vi "TCP.IP Client for Ripple Detection - Copy 5.vi"() -> ()   [LabVIEW 2021]
doc: "Demonstrates how to open a connection to an TCP server, read the data being sent, and display the data on a chart. This VI is designed to stop if the TCP connection is terminated."
uses:
  <vilib>/Utility/file.llb/Write To Spreadsheet File (string).vi
  <vilib>/Utility/file.llb/Write Delimited Spreadsheet (DBL).vi
  <vilib>/Utility/file.llb/Write To Spreadsheet File (DBL).vi
panel:
  in  "Header Info":string[][](table)=[["Test Name", "Operator", "UUT"], ["Voltage Test", "Nigel", "AAA123"]]
  in  "File Name":path=path "C:/Documents and Settings/husmith/Desktop/CSVdata.csv"
  in  "Channel Names":string[](array[string])=["Channel 1", "Channel 2", "Channel 3", "Channel 4", "Channel 5"]
  out "Filtered":dbl[](graph)
  out "Array Size 3":u32
  out "Delayed RMS2>RMS1 for 3 data":dynamicdata(graph)
  out "RMS2>RMS1 for 3 data":dynamicdata(graph)
  out "Array Size":u32
  out "RMS2>RMS1":dynamicdata(graph)
  out "RMS1":dynamicdata(graph)
  out "RMS2":dynamicdata(graph)
  out "Raw Data Collected":dynamicdata(graph)
  in  "Boolean":bool
  in  "Server Closed":string="The server VI closed the connection."
  out "Raw Data":dbl[](graph)
  in  "Stop":bool
  # "Overview: Demonstrates the use of the TCP functions to connect to a TCP server VI and receive data.\nInstructions:\n1. Ensure Simple TCP - Server.vi is already running.\n2. Run the VI.\n3. Click Stop to stop the VI. Note that if you stop the server VI, this VI will stop automatically."
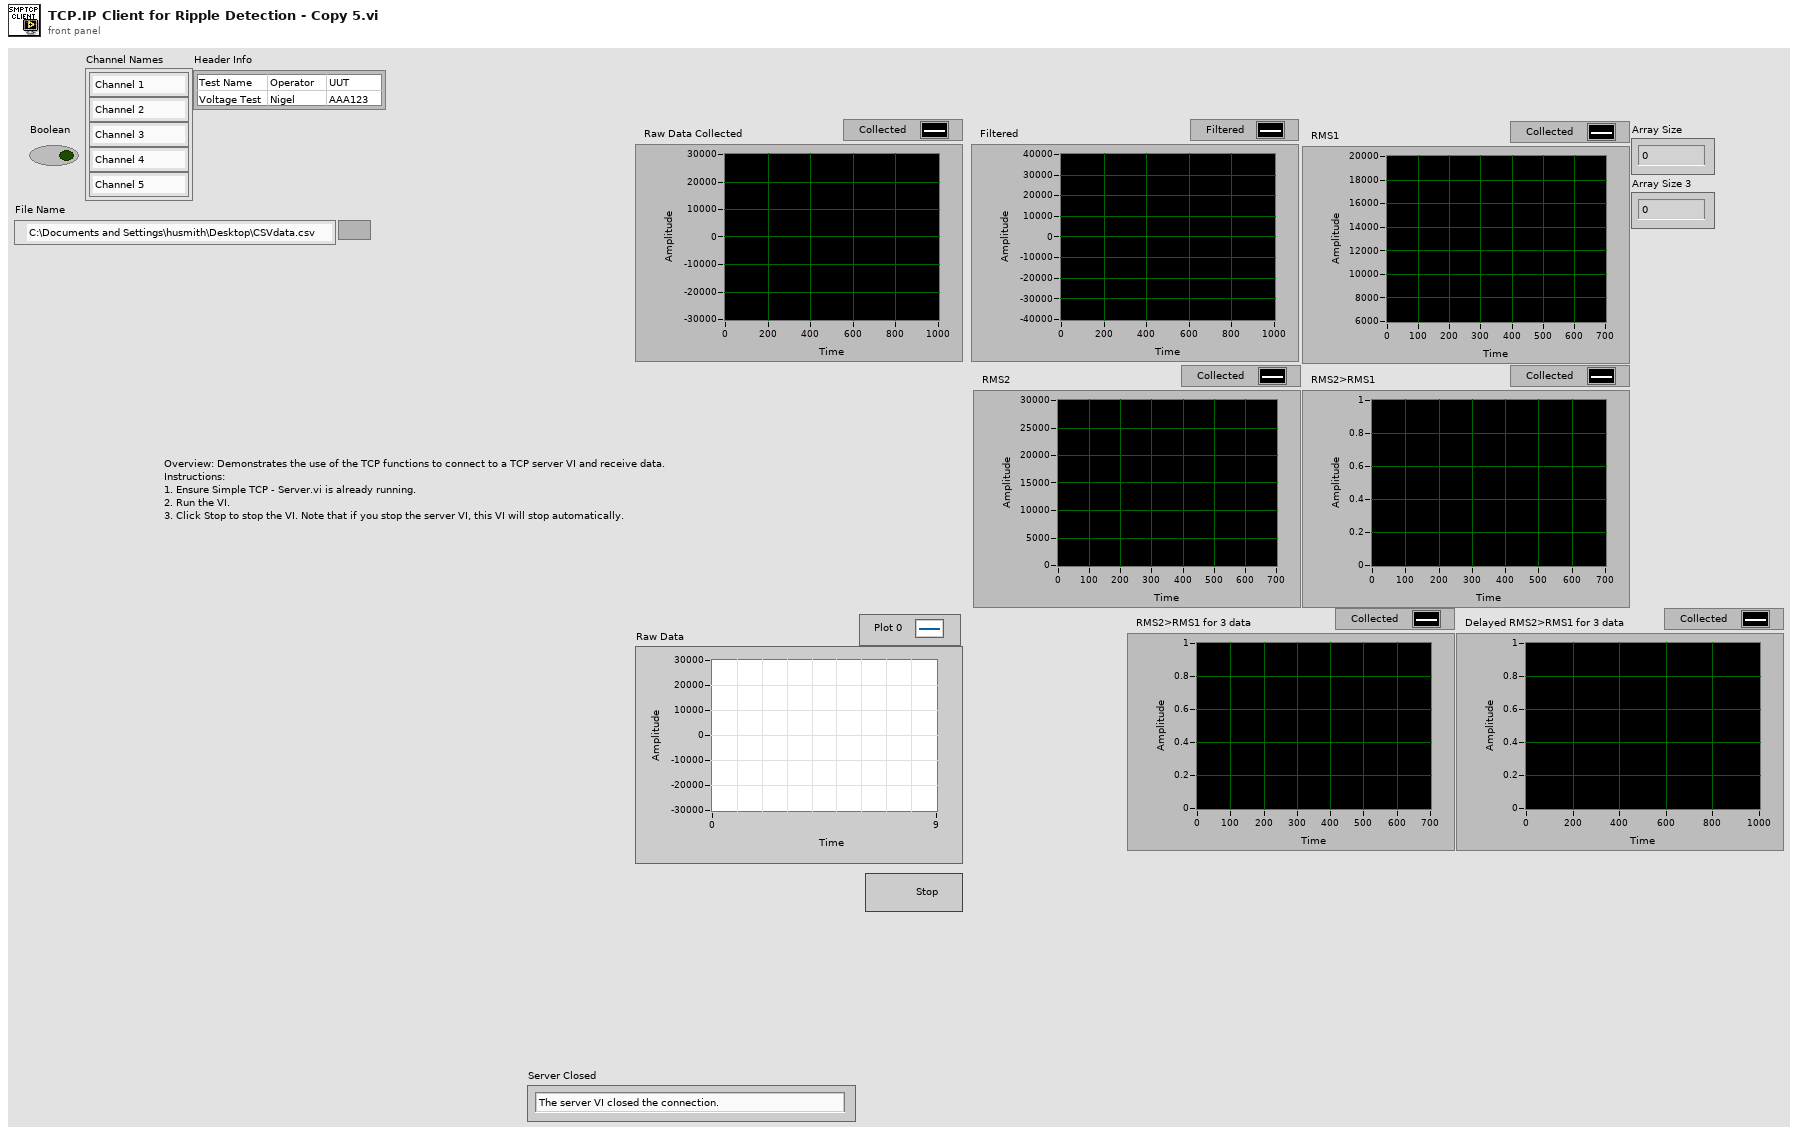
[diagram p1: front panel]
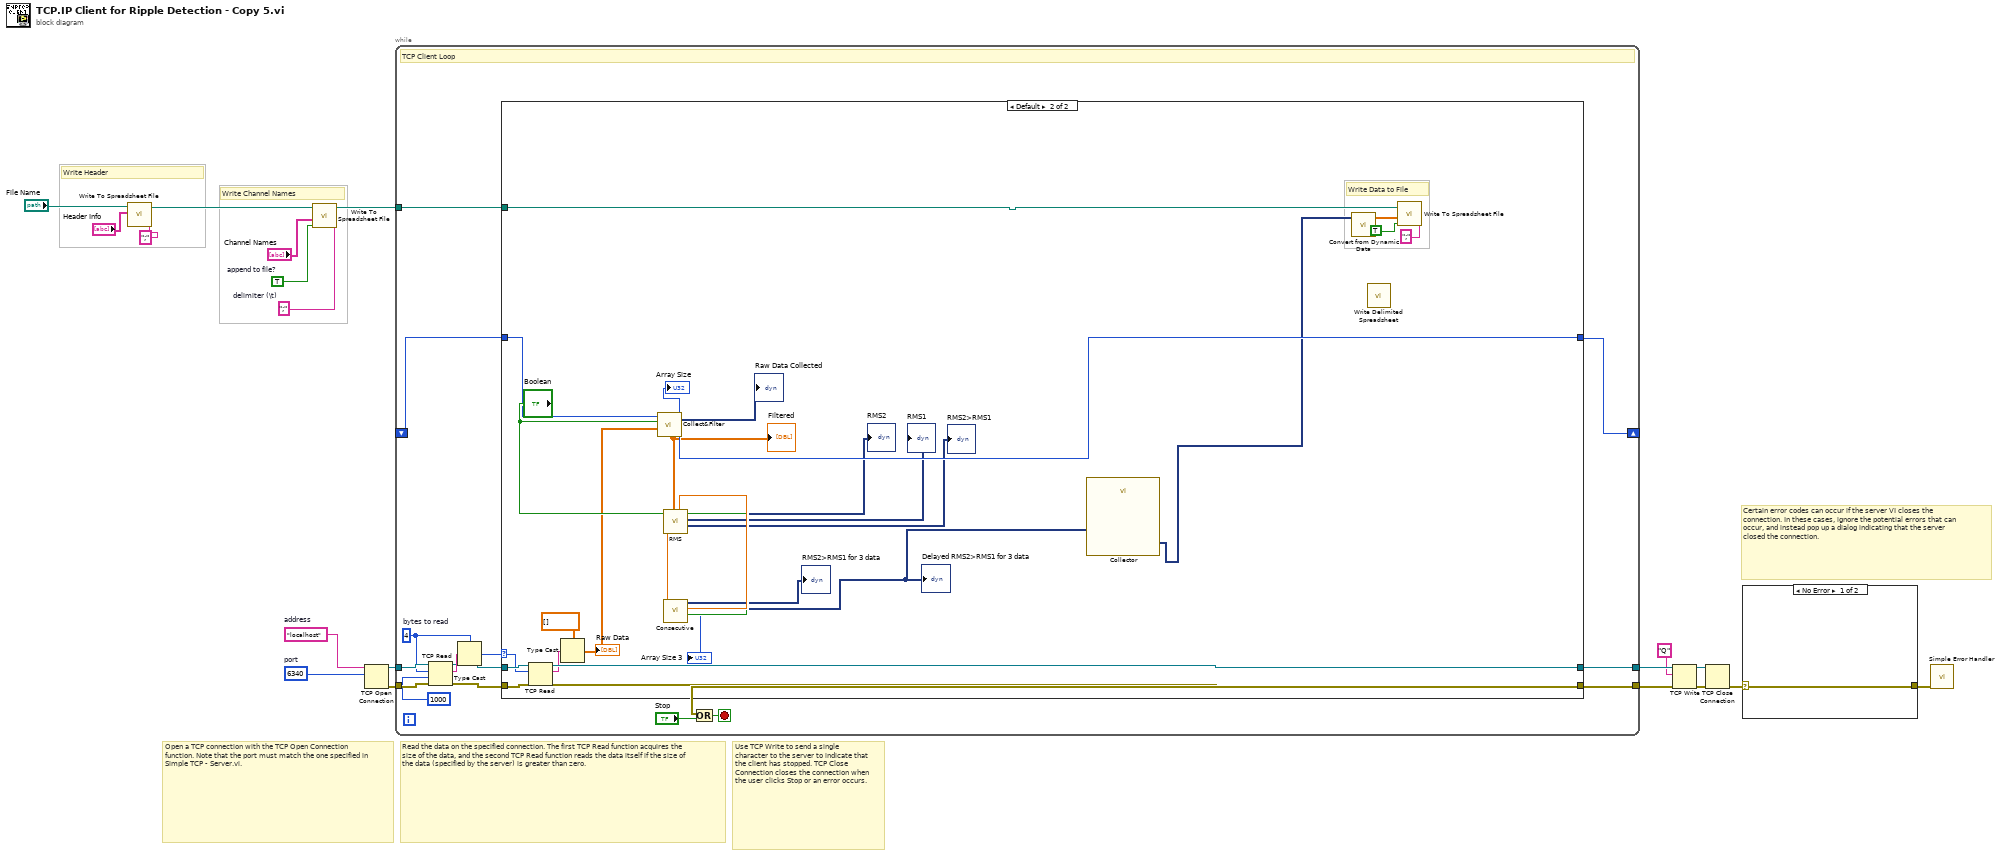
[diagram p0: block diagram]
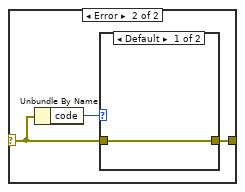
[diagram p2: hidden frame]
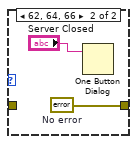
[diagram p3: hidden frame]
diagram:
  w2 = TRUE  # append to file?
  w3 = ";"  # delimiter (\t)
  w9 = u16 6340  # port
  w10 = "localhost"  # address
  # "Write Header"
  # "Write Channel Names"
  # "Certain error codes can occur if the server VI closes the connection. In these cases, ignore the potential errors that can occur, and instead pop up a dialog indicating that the server closed the connection."
  # "Use TCP Write to send a single character to the server to indicate that the client has stopped. TCP Close Connection closes the connection when the user clicks Stop or an error occurs."
  # "Read the data on the specified connection. The first TCP Read function acquires the size of the data, and the second TCP Read function reads the data itself if the size of the data (specified by the server) is greater than zero."
  # "Open a TCP connection with the TCP Open Connection function. Note that the port must match the one specified in Simple TCP - Server.vi."
  n1 = call-poly <vilib>:"Write To Spreadsheet File.vi"("delimiter (\\t)"=";" ("delimiter (\\t)"), "2D data"="Header Info", "file path (dialog if empty)"="File Name") -> ("new file path (Not A Path if cancelled)"=w7:path)  [unwired: 4 in, 1 out]
  n2 = call-poly <vilib>:"Write To Spreadsheet File.vi"("delimiter (\\t)"=w3, "append to file? (new file:F)"=w2, "1D data"="Channel Names", "file path (dialog if empty)"=w7) -> ("new file path (Not A Path if cancelled)"=w1:path)  [unwired: 3 in, 1 out]
  n3 = TCP Open Connection(address=w10, remote port or service name=w9) -> (connection ID=w19:refnum<k5>, error out=w18:errorcluster)  [unwired: 3 in]
  n4 = while {
    tunnel: w18 -> [w30]
    tunnel: w19 -> [w31]
    tunnel: [w26] -> w16
    tunnel: [w25] -> w14
    shift-right: [w21] -> _
    shift-left: _ -> [w22]
    tunnel: w1 -> [w20]
    stop <- w27 stop-if-true
    w29 = 4  # bytes to read
    # "TCP Client Loop"
    n5 = TCP Read(connection ID=w31, bytes to read=w29, error in (no error)=w30, 9:1000 ("timeout ms (25000)")) -> (connection ID out=w33:refnum<k5>, data out=w34:string, error out=w32:errorcluster)  [unwired: 1 in]
    n6 = Type Cast(type=w29, x=w34) -> (*(type *) &x=w24:i32)
    n7 = case shown="Default" w24 {
      selector: w24 -> [_ w58]
      tunnel: w33 -> [w37 w64]
      tunnel: w32 -> [w36 w63]
      tunnel: [w37 w61] -> w26
      tunnel: [w36 w60] -> w25
      tunnel: w22 -> [w35 w53]
      tunnel: [w35 w52] -> w21
      tunnel: w20 -> [_ w40]
      frame ..0 {
        # "The server has not written any data"
      }
      frame Default {
        # "Write Data to File"
        n8 = TCP Read(connection ID=w64, bytes to read=w58, error in (no error)=w63) -> (connection ID out=w61:refnum<k5>, data out=w59:string, error out=w60:errorcluster)  [unwired: 2 in]
        n9 = Type Cast(type=dbl[] [] ("chart"), x=w59) -> (*(type *) &x=w51:dbl[])
        "Raw Data" <- w51
        n10 = call "Collect&Filter.vi"("chart"=w51, "Boolean"="Boolean", "Numeric in"=w53) -> ("Collected Signals"=→"Raw Data Collected":dynamicdata, "Numeric out"=w52:i32, "Array Size"=→"Array Size":u32, "Filtered X"=w44:dbl[])  [unwired: 5 in]
        "Filtered" <- w44
        n11 = call "RMS.vi"("Filtered X"=w44) -> ("RMS2>RMS1"=→"RMS2>RMS1":dynamicdata, "RMS1"=→"RMS1":dynamicdata, "RMS2"=→"RMS2":dynamicdata, "rms value 2"=w56:dbl, "rms value"=w55:dbl)  [unwired: 6 in]
        n12 = call "Consecutive.vi"("Boolean"="Boolean", "rms value"=w55, "rms value 2"=w56) -> ("Array Size 3"=→"Array Size 3":u32, "Delayed RMS2>RMS1 for 3 data"=w38:dynamicdata, "RMS2>RMS1 for 3 data"=→"RMS2>RMS1 for 3 data":dynamicdata)  [unwired: 6 in]
        "Delayed RMS2>RMS1 for 3 data" <- w38
        n13 = call "Collector"("Signals"=w38) -> ("Collected Signals"=w39:dynamicdata)  [unwired: 9 in, 1 out]
        n14 = call "Convert from Dynamic Data"("Dynamic Data Type"=w39) -> ("Array"=w41:dbl[])  [unwired: 3 in]
        n15 = call-poly <vilib>:"Write Delimited Spreadsheet.vi"() -> ()  [unwired: 14 in, 2 out]
        n16 = call-poly <vilib>:"Write To Spreadsheet File.vi"("delimiter (\\t)"=";" ("delimiter (\\t)"), "append to file? (new file:F)"=TRUE, "1D data"=w41, "file path (dialog if empty)"=w40) -> ()  [unwired: 3 in, 2 out]
      }
    }
    n17 = Or(x=w25, y="Stop") -> (x .or. y?=w27:bool)
  }
  n18 = TCP Write(connection ID=w16, data in="Q", error in (no error)=w14) -> (connection ID out=w17:refnum<k5>, error out=w15:errorcluster)  [unwired: 2 out]
  n19 = TCP Close Connection(connection ID=w17, error in (no error)=w15) -> (error out=w12:errorcluster)  [unwired: 1 in, 1 out]
  n20 = case shown="No Error" w12 {
    selector: w12 -> [w65 w67]
    tunnel: [w65 w66] -> w11
    frame No Error {
    }
    frame Error {
      n21 = Unbundle By Name(w67) -> ("code"=w68:i32)
      n22 = case shown="Default" w68 {
        tunnel: w67 -> [w69 _]
        tunnel: [w69 w71] -> w66
        frame Default {
        }
        frame 62, 64, 66 {
          w71 = errorcluster {"status"=FALSE, "code"=0, "source"=""}  # No error
          n23 = One Button Dialog(message="Server Closed") -> ()  [unwired: 1 in, 1 out]
        }
      }
    }
  }
  n24 = call <vilib>:"Simple Error Handler.vi"("error in (no error)"=w11) -> ()  [unwired: 4 in, 5 out]
